vi "Read Spectra.vi"(8 "error in (no error)":errorcluster, 11 "VISA resource name":refnum<visa-resource-name>) -> (0 "error out":errorcluster, 2 "Spectrum by Pixels":dbl[](array[numeric]), 3 "VISA resource name out":refnum<visa-resource-name>)   [LabVIEW 2021, in "Ocean Optics 2000 4000.lvlib"]
doc: "Reads the full spectra from the spectrometer. The spectrum is displayed in an array according to the pixel number."
uses:
  <instrlib>/Ocean Optics 2000 4000/Ocean Optics 2000 4000.lvlib
panel:
  # "Note:\nThis VI has been obsoleted from the driver and is included for compatibility with existing applications New applications should use the Read Spectrum VI.  \nNew applications should use the Read Spectrum VI."
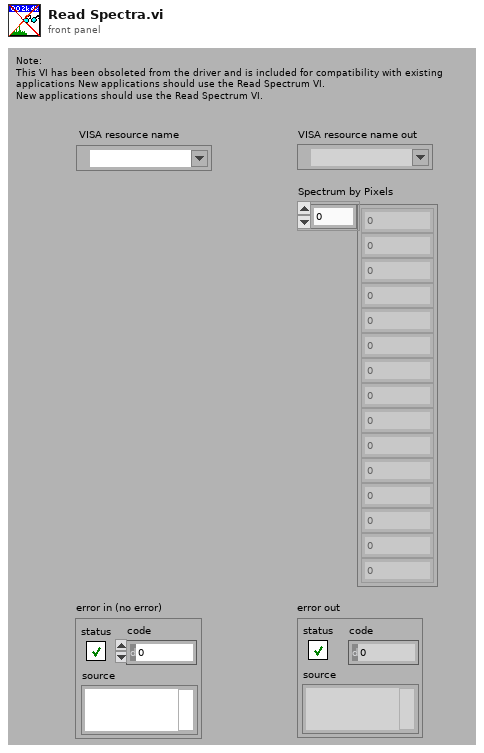
[diagram p1: front panel]
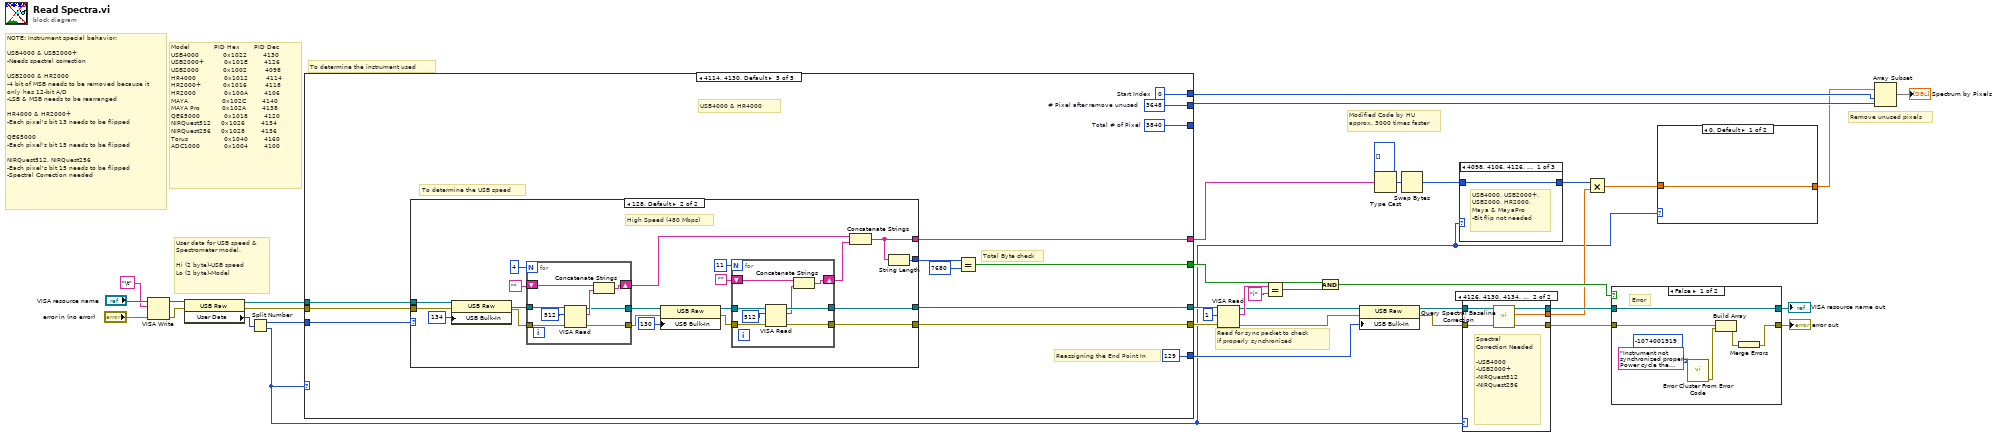
[diagram p0: block diagram]
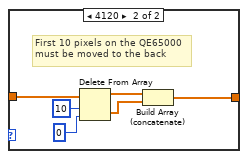
[diagram p2: hidden frame]
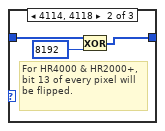
[diagram p3: hidden frame]
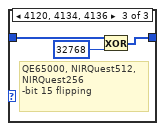
[diagram p4: hidden frame]
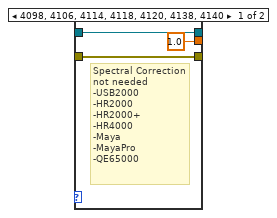
[diagram p5: hidden frame]
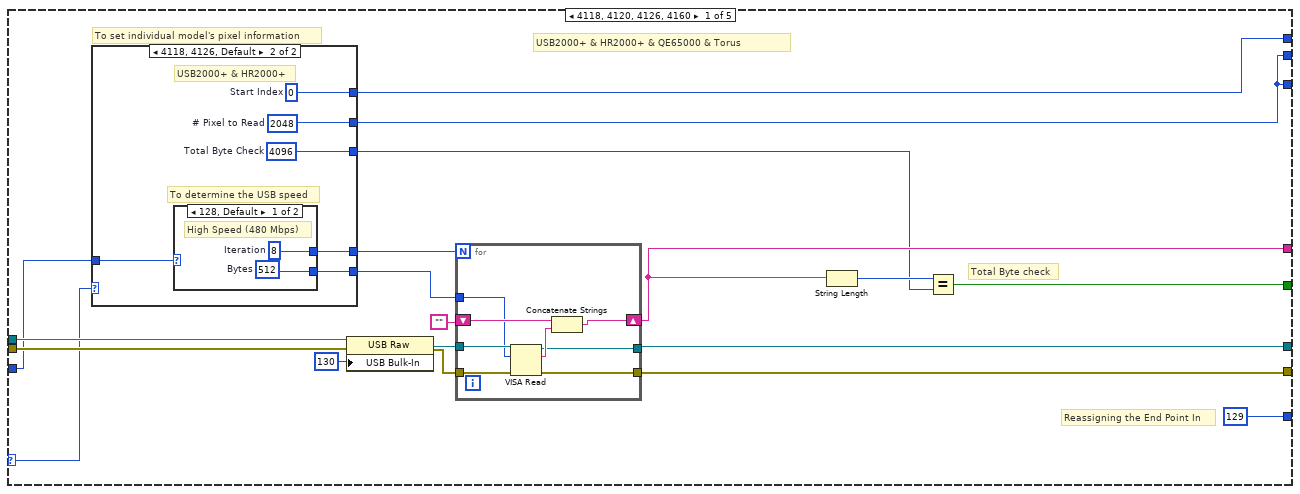
[diagram p6: hidden frame]
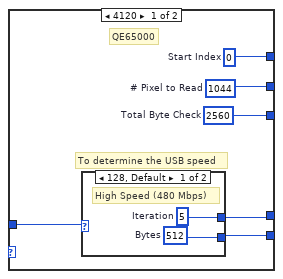
[diagram p7: hidden frame]
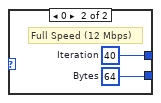
[diagram p8: hidden frame]
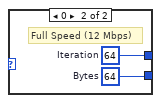
[diagram p9: hidden frame]
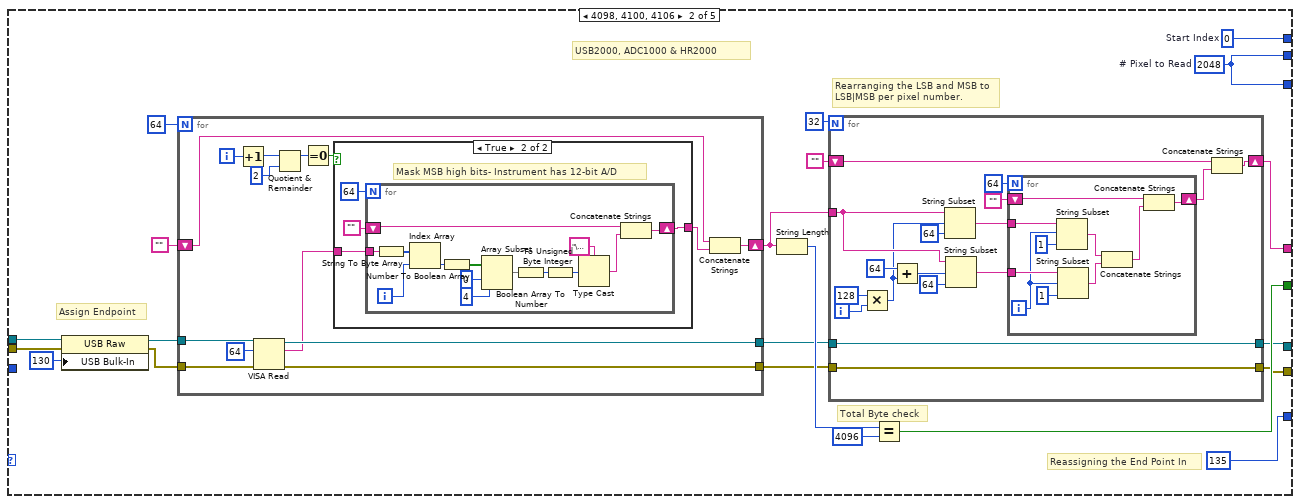
[diagram p10: hidden frame]
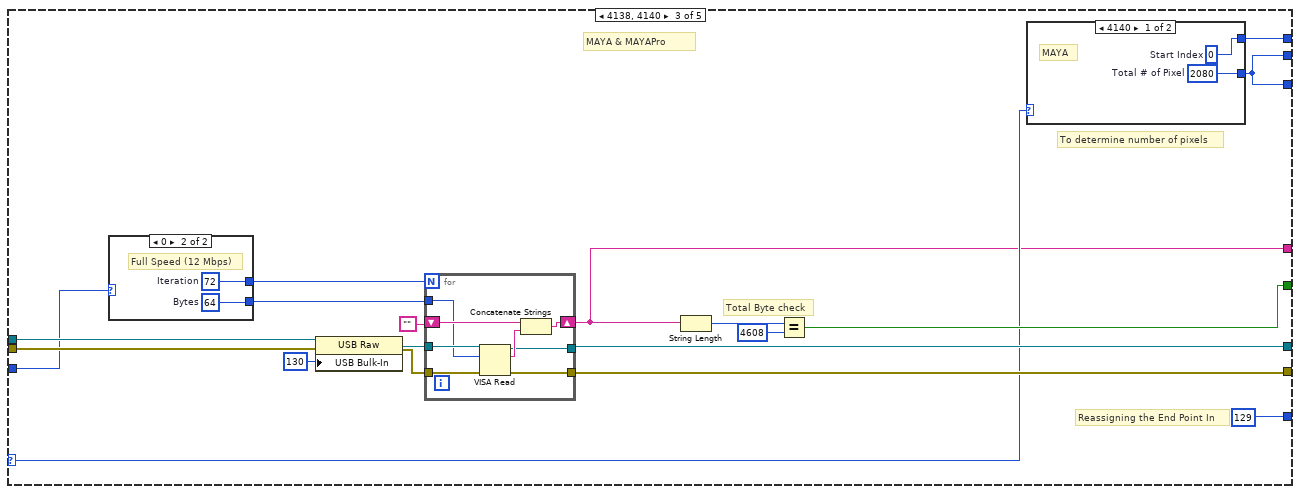
[diagram p12: hidden frame]
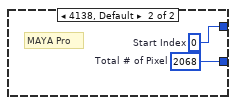
[diagram p13: hidden frame]
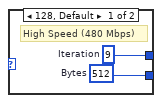
[diagram p14: hidden frame]
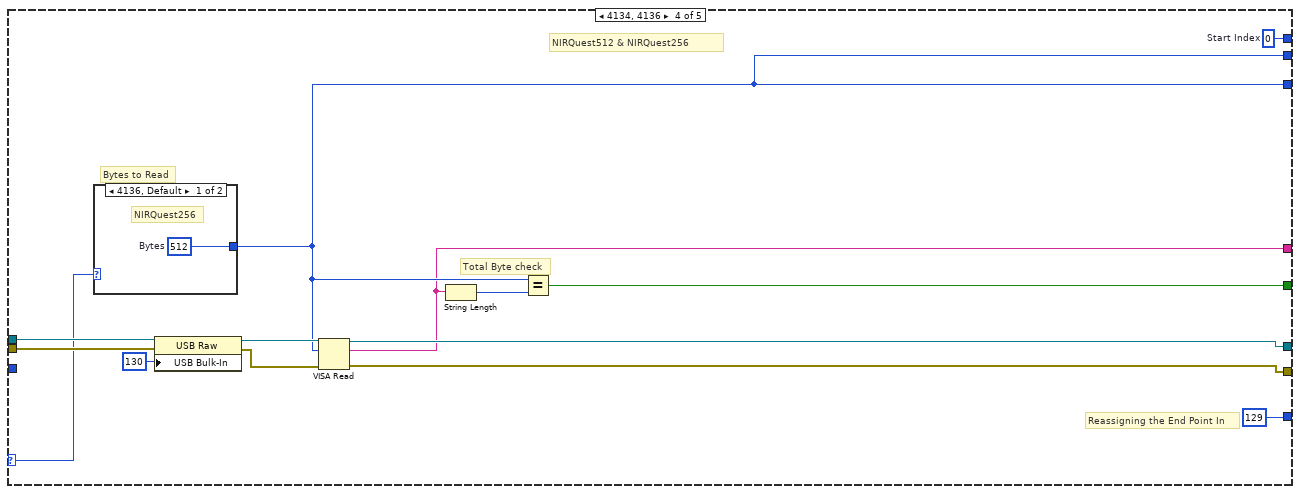
[diagram p15: hidden frame]
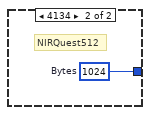
[diagram p16: hidden frame]
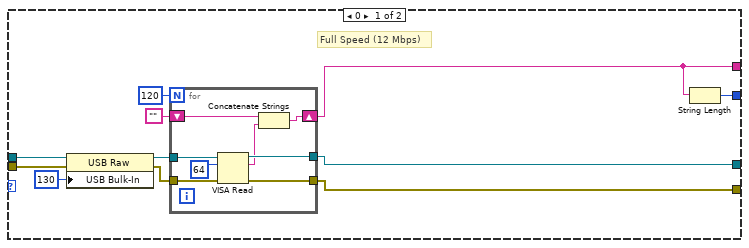
[diagram p17: hidden frame]
diagram:
  # "Model            PID Hex       PID Dec \nUSB4000            0x1022        4130 \nUSB2000+          0x101E        4126 \nUSB2000            0x1002         4098\nHR4000              0x1012         4114\nHR2000+           0x1016         4118\nHR2000              0x100A        4106\nMAYA                 0x102C        4140\nMAYA Pro           0x102A        4138\nQE65000            0x1018        4120\nNIRQuest512     0x1026        4134\nNIRQuest256     0x1028        4136\nTorus                  0x1040        4160\nADC1000            0x1004        4100"
  # "Modified Code by HU\napprox. 3000 times faster"
  # "NOTE: Instrument special behavior:\n\nUSB4000 & USB2000+ \n-Needs spectral correction\n\nUSB2000 & HR2000\n-4 bit of MSB needs to be removed because it only has 12-bit A/D\n-LSB & MSB needs to be rearranged \n\nHR4000 & HR2000+\n-Each pixel's bit 13 needs to be flipped\n\nQE65000\n-Each pixel's bit 15 needs to be flipped\n\nNIRQuest512, NIRQuest256\n-Each pixel's bit 15 needs to be flipped\n-Spectral Correction needed"
  # "Read for sync packet to check \nif properly synchronized"
  # "User data for USB speed & Spectrometer model. \n\nHi (2 byte)-USB speed\nLo (2 byte)-Model"
  # "To determine the instrument used"
  # "Remove unused pixels"
  n1 = VISA Write(VISA resource name="VISA resource name", write buffer="\t", error in (no error)="error in (no error)") -> (VISA resource name out=w34:refnum<visa-resource-name>, error out=w35:errorcluster)  [unwired: 1 out]
  n2 = property class="USB Raw"(reference=w34, error in=w35) -> (reference out=w33:refnum<visa-resource-name>, error out=w32:errorcluster, "User Data"=w15:u32)
  n3 = Split Number(x=w15) -> (hi(x)=w14:u16, lo(x)=w4:u16)
  n4 = case shown="4114, 4130, Default" w4 {
    selector: w4 -> [w42 _ w171 w210 _]
    tunnel: w33 -> [w56 w105 w185 w212 w230]
    tunnel: w32 -> [w57 w104 w184 w211 w229]
    tunnel: [w55 w86 w168 w203 w219] -> w9
    tunnel: [w54 w89 w183 w207 w228] -> w30
    tunnel: [w53 w87 w182 w206 w227] -> w29
    tunnel: [w52 w97 w179 w208 w223] -> w13
    tunnel: w14 -> [w45 _ w174 _ w226]
    tunnel: [w40 w96 w169 w205 w222] -> _
    tunnel: [w40 w96 w169 w205 w221] -> w12
    tunnel: [w41 w95 w170 w204 w220] -> w11
    tunnel: [i16 129 ("USB Settings:Bulk-In Pipe") i16 135 ("USB Settings:Bulk-In Pipe") i16 129 ("USB Settings:Bulk-In Pipe") i16 129 ("USB Settings:Bulk-In Pipe") i16 129 ("USB Settings:Bulk-In Pipe")] -> w10
    frame 4118, 4120, 4126, 4160 {
      # "To set individual model's pixel information"
      # "Total Byte check"
      # "Reassigning the End Point In"
      # "USB2000+ & HR2000+ & QE65000 & Torus"
      n5 = case shown="4118, 4126, Default" w42 {
        tunnel: w45 -> [w63 w73]
        tunnel: [w62 w72] -> w44
        tunnel: [w61 w71] -> w43
        tunnel: [w60 w70] -> w41
        tunnel: [w59 w69] -> w40
        tunnel: [w58 w68] -> w39
        frame 4120 {
          w58 = 2560  # Total Byte Check
          w60 = 0  # Start Index
          w59 = 1044  # # Pixel to Read
          # "To determine the USB speed"
          # "QE65000"
          n6 = case shown="128, Default" w63 {
            tunnel: [w65 w67] -> w62
            tunnel: [w64 w66] -> w61
            frame 128, Default {
              w64 = u32 512  # Bytes
              w65 = 5  # Iteration
              # "High Speed (480 Mbps)"
            }
            frame 0 {
              w66 = u32 64  # Bytes
              w67 = 40  # Iteration
              # "Full Speed (12 Mbps)"
            }
          }
        }
        frame 4118, 4126, Default {
          w68 = 4096  # Total Byte Check
          w70 = 0  # Start Index
          w69 = 2048  # # Pixel to Read
          # "USB2000+ & HR2000+"
          # "To determine the USB speed"
          n7 = case shown="128, Default" w73 {
            tunnel: [w75 w77] -> w72
            tunnel: [w74 w76] -> w71
            frame 128, Default {
              w74 = u32 512  # Bytes
              w75 = 8  # Iteration
              # "High Speed (480 Mbps)"
            }
            frame 0 {
              w76 = u32 64  # Bytes
              w77 = 64  # Iteration
              # "Full Speed (12 Mbps)"
            }
          }
        }
      }
      n8 = property class="USB Raw"(reference=w56, error in=w57, "USB Bulk-In"=i16 130 ("USB Settings:Bulk-In Pipe")) -> (reference out=w48:refnum<visa-resource-name>, error out=w47:errorcluster)
      n9 = for {
        N: w44 -> [_]
        tunnel: w48 -> [w85]
        tunnel: w47 -> [w84]
        shift-right: [w83] -> w55
        shift-left: "" -> [w82]
        tunnel: [w80] -> w54
        tunnel: [w79] -> w53
        tunnel: w43 -> [w78]
        n10 = VISA Read(VISA resource name=w85, byte count=w78, error in (no error)=w84) -> (VISA resource name out=w80:refnum<visa-resource-name>, read buffer=w81:string, error out=w79:errorcluster)  [unwired: 1 out]
        n11 = Concatenate Strings(w82, w81) -> (w83:string)
      }
      n12 = String Length(string=w55) -> (length=w51:i32)
      n13 = Equal?(x=w51, y=w39) -> (x = y?=w52:bool)
    }
    frame 4098, 4100, 4106 {
      w95 = 0  # Start Index
      w96 = 2048  # # Pixel to Read
      # "Total Byte check"
      # "Reassigning the End Point In"
      # "Assign Endpoint"
      # "Rearranging the LSB and MSB to LSB|MSB per pixel number."
      # "USB2000, ADC1000 & HR2000"
      n14 = property class="USB Raw"(reference=w105, error in=w104, "USB Bulk-In"=i16 130 ("USB Settings:Bulk-In Pipe")) -> (reference out=w101:refnum<visa-resource-name>, error out=w100:errorcluster)
      n15 = for {
        N: 64 -> [_]
        tunnel: w101 -> [w147]
        tunnel: w100 -> [w146]
        shift-right: [w136] -> w91
        shift-left: "" -> [w134]
        tunnel: [w144] -> w90
        tunnel: [w143] -> w88
        i -> [w142]
        n16 = Increment(x=w142) -> (x+1=w141:i32)
        n17 = VISA Read(VISA resource name=w147, byte count=u32 64, error in (no error)=w146) -> (VISA resource name out=w144:refnum<visa-resource-name>, read buffer=w137:string, error out=w143:errorcluster)  [unwired: 1 out]
        n18 = Quotient & Remainder(x=w141, y=2) -> (x-y*floor(x/y)=w139:i32)  [unwired: 1 out]
        n19 = Equal To 0?(x=w139) -> (x = 0?=w138:bool)
        n20 = case shown="True" w138 {
          tunnel: w137 -> [w148 w152]
          tunnel: [w148 w150] -> w135
          frame False {
            # "LSB- Not masked"
          }
          frame True {
            # "Mask MSB high bits- Instrument has 12-bit A/D"
            n21 = for {
              N: 64 -> [_]
              tunnel: w152 -> [w166]
              shift-right: [w156] -> w150
              shift-left: "" -> [w157]
              i -> [w158]
              n22 = String To Byte Array(string=w166) -> (unsigned byte array=w165:u8[])
              n23 = Index Array(array=w165, index=w158) -> (element=w164:u8)
              n24 = Number To Boolean Array(number=w164) -> (Boolean array=w163:bool[])
              n25 = Array Subset(array=w163, index=0, length=4) -> (w160:bool[])
              n26 = Boolean Array To Number(Boolean array=w160) -> (number=w154:u32)
              n27 = To Unsigned Byte Integer(number=w154) -> (unsigned 8bit integer=w153:u8)
              n28 = Type Cast(type="\u0000", x=w153) -> (*(type *) &x=w155:string)
              n29 = Concatenate Strings(w157, w155) -> (w156:string)
            }
          }
        }
        n30 = Concatenate Strings(w134, w135) -> (w136:string)
      }
      n31 = String Length(string=w91) -> (length=w99:i32)
      n32 = for {
        N: 32 -> [_]
        tunnel: w91 -> [w123]
        shift-right: [w114] -> w86
        shift-left: "" -> [w112]
        tunnel: w90 -> [w108]
        tunnel: [w108] -> w89
        tunnel: w88 -> [w107]
        tunnel: [w107] -> w87
        i -> [w111]
        n33 = Multiply(x=128, y=w111) -> (x*y=w109:i32)
        n34 = Add(x=64, y=w109) -> (x+y=w120:i32)
        n35 = String Subset(string=w123, offset (0)=w109, length (rest)=64 ("length (rest)")) -> (substring=w117:string)
        n36 = String Subset(string=w123, offset (0)=w120, length (rest)=64 ("length (rest)")) -> (substring=w116:string)
        n37 = for {
          N: 64 -> [_]
          tunnel: w117 -> [w133]
          tunnel: w116 -> [w132]
          shift-right: [w125] -> w113
          shift-left: "" -> [w126]
          i -> [w129]
          n38 = String Subset(string=w133, offset (0)=w129, length (rest)=1 ("length (rest)")) -> (substring=w128:string)
          n39 = String Subset(string=w132, offset (0)=w129, length (rest)=1 ("length (rest)")) -> (substring=w127:string)
          n40 = Concatenate Strings(w128, w127) -> (w124:string)
          n41 = Concatenate Strings(w126, w124) -> (w125:string)
        }
        n42 = Concatenate Strings(w112, w113) -> (w114:string)
      }
      n43 = Equal?(x=w99, y=4096) -> (x = y?=w97:bool)
    }
    frame 4138, 4140 {
      # "To determine number of pixels"
      # "Reassigning the End Point In"
      # "Total Byte check"
      # "MAYA & MAYAPro"
      n44 = case shown="0" w174 {
        tunnel: [w191 w193] -> w173
        tunnel: [w190 w192] -> w172
        frame 128, Default {
          w190 = u32 512  # Bytes
          w191 = 9  # Iteration
          # "High Speed (480 Mbps)"
        }
        frame 0 {
          w192 = u32 64  # Bytes
          w193 = 72  # Iteration
          # "Full Speed (12 Mbps)"
        }
      }
      n45 = property class="USB Raw"(reference=w185, error in=w184, "USB Bulk-In"=i16 130 ("USB Settings:Bulk-In Pipe")) -> (reference out=w177:refnum<visa-resource-name>, error out=w176:errorcluster)
      n46 = for {
        N: w173 -> [_]
        tunnel: w177 -> [w201]
        tunnel: w176 -> [w200]
        shift-right: [w199] -> w168
        shift-left: "" -> [w198]
        tunnel: [w196] -> w183
        tunnel: [w195] -> w182
        tunnel: w172 -> [w194]
        n47 = VISA Read(VISA resource name=w201, byte count=w194, error in (no error)=w200) -> (VISA resource name out=w196:refnum<visa-resource-name>, read buffer=w197:string, error out=w195:errorcluster)  [unwired: 1 out]
        n48 = Concatenate Strings(w198, w197) -> (w199:string)
      }
      n49 = String Length(string=w168) -> (length=w180:i32)
      n50 = Equal?(x=w180, y=4608) -> (x = y?=w179:bool)
      n51 = case shown="4140" w171 {
        tunnel: [w186 w189] -> w170
        tunnel: [w187 w188] -> w169
        frame 4140 {
          w187 = 2080  # Total # of Pixel
          w186 = 0  # Start Index
          # "MAYA"
        }
        frame 4138, Default {
          w188 = 2068  # Total # of Pixel
          w189 = 0  # Start Index
          # "MAYA Pro"
        }
      }
    }
    frame 4134, 4136 {
      w204 = 0  # Start Index
      # "Reassigning the End Point In"
      # "Bytes to Read"
      # "Total Byte check"
      # "NIRQuest512 & NIRQuest256"
      n52 = case shown="4136, Default" w210 {
        tunnel: [w216 w217] -> w205
        frame 4136, Default {
          w216 = u32 512  # Bytes
          # "NIRQuest256"
        }
        frame 4134 {
          w217 = u32 1024  # Bytes
          # "NIRQuest512"
        }
      }
      n53 = property class="USB Raw"(reference=w212, error in=w211, "USB Bulk-In"=i16 130 ("USB Settings:Bulk-In Pipe")) -> (reference out=w214:refnum<visa-resource-name>, error out=w213:errorcluster)
      n54 = VISA Read(VISA resource name=w214, byte count=w205, error in (no error)=w213) -> (VISA resource name out=w207:refnum<visa-resource-name>, read buffer=w203:string, error out=w206:errorcluster)  [unwired: 1 out]
      n55 = String Length(string=w203) -> (length=w209:i32)
      n56 = Equal?(x=w205, y=w209) -> (x = y?=w208:bool)
    }
    frame 4114, 4130, Default {
      w220 = 0  # Start Index
      w221 = 3648  # # Pixel after remove unused
      w222 = 3840  # Total # of Pixel
      # "Reassigning the End Point In"
      # "Total Byte check"
      # "To determine the USB speed"
      # "USB4000 & HR4000"
      n57 = case shown="128, Default" w226 {
        tunnel: w230 -> [w236 w269]
        tunnel: w229 -> [w235 w268]
        tunnel: [w234 w254] -> w228
        tunnel: [w233 w253] -> w227
        tunnel: [w231 w252] -> w219
        tunnel: [w232 w251] -> w224
        frame 0 {
          # "Full Speed (12 Mbps)"
          n58 = property class="USB Raw"(reference=w236, error in=w235, "USB Bulk-In"=i16 130 ("USB Settings:Bulk-In Pipe")) -> (reference out=w240:refnum<visa-resource-name>, error out=w237:errorcluster)
          n59 = for {
            N: 120 -> [_]
            tunnel: w240 -> [w248]
            tunnel: w237 -> [w247]
            tunnel: [w246] -> w234
            tunnel: [w245] -> w233
            shift-right: [w244] -> w231
            shift-left: "" -> [w243]
            n60 = VISA Read(VISA resource name=w248, byte count=u32 64, error in (no error)=w247) -> (VISA resource name out=w246:refnum<visa-resource-name>, read buffer=w242:string, error out=w245:errorcluster)  [unwired: 1 out]
            n61 = Concatenate Strings(w243, w242) -> (w244:string)
          }
          n62 = String Length(string=w231) -> (length=w232:i32)
        }
        frame 128, Default {
          # "High Speed (480 Mbps)"
          n63 = property class="USB Raw"(reference=w269, error in=w268, "USB Bulk-In"=i16 134 ("USB Settings:Bulk-In Pipe")) -> (reference out=w266:refnum<visa-resource-name>, error out=w265:errorcluster)
          n64 = for {
            N: 4 -> [_]
            tunnel: w266 -> [w277]
            tunnel: w265 -> [w276]
            shift-right: [w274] -> w250
            shift-left: "" -> [w273]
            tunnel: [w271] -> w259
            tunnel: [w270] -> w258
            n65 = VISA Read(VISA resource name=w277, byte count=u32 512, error in (no error)=w276) -> (VISA resource name out=w271:refnum<visa-resource-name>, read buffer=w272:string, error out=w270:errorcluster)  [unwired: 1 out]
            n66 = Concatenate Strings(w273, w272) -> (w274:string)
          }
          n67 = property class="USB Raw"(reference=w259, error in=w258, "USB Bulk-In"=i16 130 ("USB Settings:Bulk-In Pipe")) -> (reference out=w263:refnum<visa-resource-name>, error out=w256:errorcluster)
          n68 = for {
            N: 11 -> [_]
            tunnel: w263 -> [w284]
            tunnel: w256 -> [w283]
            tunnel: [w282] -> w254
            tunnel: [w281] -> w253
            shift-right: [w280] -> w255
            shift-left: "" -> [w279]
            n69 = VISA Read(VISA resource name=w284, byte count=u32 512, error in (no error)=w283) -> (VISA resource name out=w282:refnum<visa-resource-name>, read buffer=w278:string, error out=w281:errorcluster)  [unwired: 1 out]
            n70 = Concatenate Strings(w279, w278) -> (w280:string)
          }
          n71 = Concatenate Strings(w250, w255) -> (w252:string)
          n72 = String Length(string=w252) -> (length=w251:i32)
        }
      }
      n73 = Equal?(x=w224, y=7680) -> (x = y?=w223:bool)
    }
  }
  n74 = VISA Read(VISA resource name=w30, byte count=u32 1, error in (no error)=w29) -> (VISA resource name out=w24:refnum<visa-resource-name>, read buffer=w28:string, error out=w23:errorcluster)  [unwired: 1 out]
  n75 = Equal?(x=w28, y="i") -> (x = y?=w25:bool)
  n76 = And(x=w13, y=w25) -> (x .and. y?=w26:bool)
  n77 = property class="USB Raw"(reference=w24, error in=w23, "USB Bulk-In"=w10) -> (reference out=w22:refnum<visa-resource-name>, error out=w21:errorcluster)
  n78 = Type Cast(type=u16[] [], x=w9) -> (*(type *) &x=w8:u16[])
  n79 = Swap Bytes(anything=w8) -> (byte swapped=w6:u16[])
  n80 = case shown="4098, 4106, 4126, 4130, 4138, 4140, Default" w4 {
    tunnel: w6 -> [w286 w289 w291]
    tunnel: [w286 w287 w290] -> w5
    frame 4098, 4106, 4126, 4130, 4138, 4140, Default {
      # "USB4000, USB2000+, USB2000, HR2000, Maya & MayaPro\n-Bit flip not needed"
    }
    frame 4114, 4118 {
      # "For HR4000 & HR2000+, bit 13 of every pixel will be flipped."
      n81 = Exclusive Or(1:u16 8192 ("y"), 2:w289) -> (0:w287:u16[])
    }
    frame 4120, 4134, 4136 {
      # "QE65000, NIRQuest512, NIRQuest256 \n-bit 15 flipping"
      n82 = Exclusive Or(1:u16 32768 ("y"), 2:w291) -> (0:w290:u16[])
    }
  }
  n83 = case shown="4126, 4130, 4134, 4136, Default" w4 {
    tunnel: w22 -> [w295 w300]
    tunnel: w21 -> [w294 w299]
    tunnel: [w295 w298] -> w20
    tunnel: [w294 w297] -> w19
    tunnel: [1.0 ("Spectral Baseline Correction") w296] -> w16
    frame 4098, 4106, 4114, 4118, 4120, 4138, 4140 {
      # "Spectral Correction not needed\n-USB2000\n-HR2000\n-HR2000+\n-HR4000\n-Maya\n-MayaPro\n-QE65000"
    }
    frame 4126, 4130, 4134, 4136, Default {
      # "Spectral Correction Needed\n\n-USB4000\n-USB2000+\n-NIRQuest512\n-NIRQuest256"
      n84 = call <instrlib>:"Query Spectral Baseline Correction.vi"("error in (no error)"=w299, "VISA resource name"=w300) -> ("error out"=w297:errorcluster, "Spectral Baseline Correction"=w296:dbl, "VISA resource name out"=w298:refnum<visa-resource-name>)  [unwired: 7 out]
    }
  }
  n85 = Multiply(x=w5, y=w16) -> (x*y=w3:dbl[])
  n86 = case shown="False" w26 {
    tunnel: w19 -> [w307 w309]
    tunnel: [w303 w309] -> w17
    tunnel: [w302 w308] -> w18
    tunnel: w20 -> [w302 w308]
    frame False {
      # "Error"
      n87 = call <vilib>:"Error Cluster From Error Code.vi"("error message (\"\")"="Instrument not synchronized properly. Power cycle the instrument." ("error message (\"\")"), "error code (0)"=-1074001919 ("code")) -> ("error out"=w304:errorcluster)  [unwired: 2 in, 5 out]
      n88 = Build Array(w307, w304) -> (w301:errorcluster[])
      n89 = Merge Errors(w301) -> (w303:errorcluster)
    }
    frame True {
      # "No error. Instrument properly synchronized."
    }
  }
  "VISA resource name out" <- w18
  "error out" <- w17
  n90 = case shown="0, Default" w4 {
    tunnel: w3 -> [w310 w316]
    tunnel: [w310 w311] -> w2
    frame 0, Default {
    }
    frame 4120 {
      # "First 10 pixels on the QE65000\nmust be moved to the back"
      n91 = Delete From Array(array=w316, length=10, index=0) -> (deleted portion=w312:dbl[], array with subset deleted=w313:dbl[])
      n92 = Build Array (concatenate)(w313, w312) -> (w311:dbl[])
    }
  }
  n93 = Array Subset(array=w2, index=w11, length=w12) -> (→"Spectrum by Pixels":dbl[])
